vi "HEWH Mixing Valve.vi"(8 "Error In":errorcluster, 10 "ERD Data Out":T4[](array[typedef]) {"ERD Number" format="%.0x"}, 11 "ERD Data":T1 {"ERD Therm Data"."EEV Possition" format="%0.0f"; "ERD Therm Data"."T6" format="%.1f"; "ERD Therm Data"."T2" format="%.1f"; "ERD Therm Data"."T3a" format="%.1f"; "ERD Therm Data"."T3b" format="%.1f"; "ERD Therm Data"."T4" format="%.1f"; "ERD Therm Data"."T5" format="%.1f"; "ERD Therm Data"."Current" format="%.1f"}) -> (0 "Error Out":errorcluster, 3 "ERD Data Out":T1 {"ERD Therm Data"."EEV Possition" format="%0.0f"; "ERD Therm Data"."T6" format="%.1f"; "ERD Therm Data"."T2" format="%.1f"; "ERD Therm Data"."T3a" format="%.1f"; "ERD Therm Data"."T3b" format="%.1f"; "ERD Therm Data"."T4" format="%.1f"; "ERD Therm Data"."T5" format="%.1f"; "ERD Therm Data"."Current" format="%.1f"})   [LabVIEW 2016]
uses:
  type defs/ERD Read Data Out.ctl
  type defs/HEWH ERD Data.ctl
  type defs/HEWH Faults.ctl
  type defs/HEWH Mixing Valve.ctl
  library/GEA2_Toolkit.lvlib
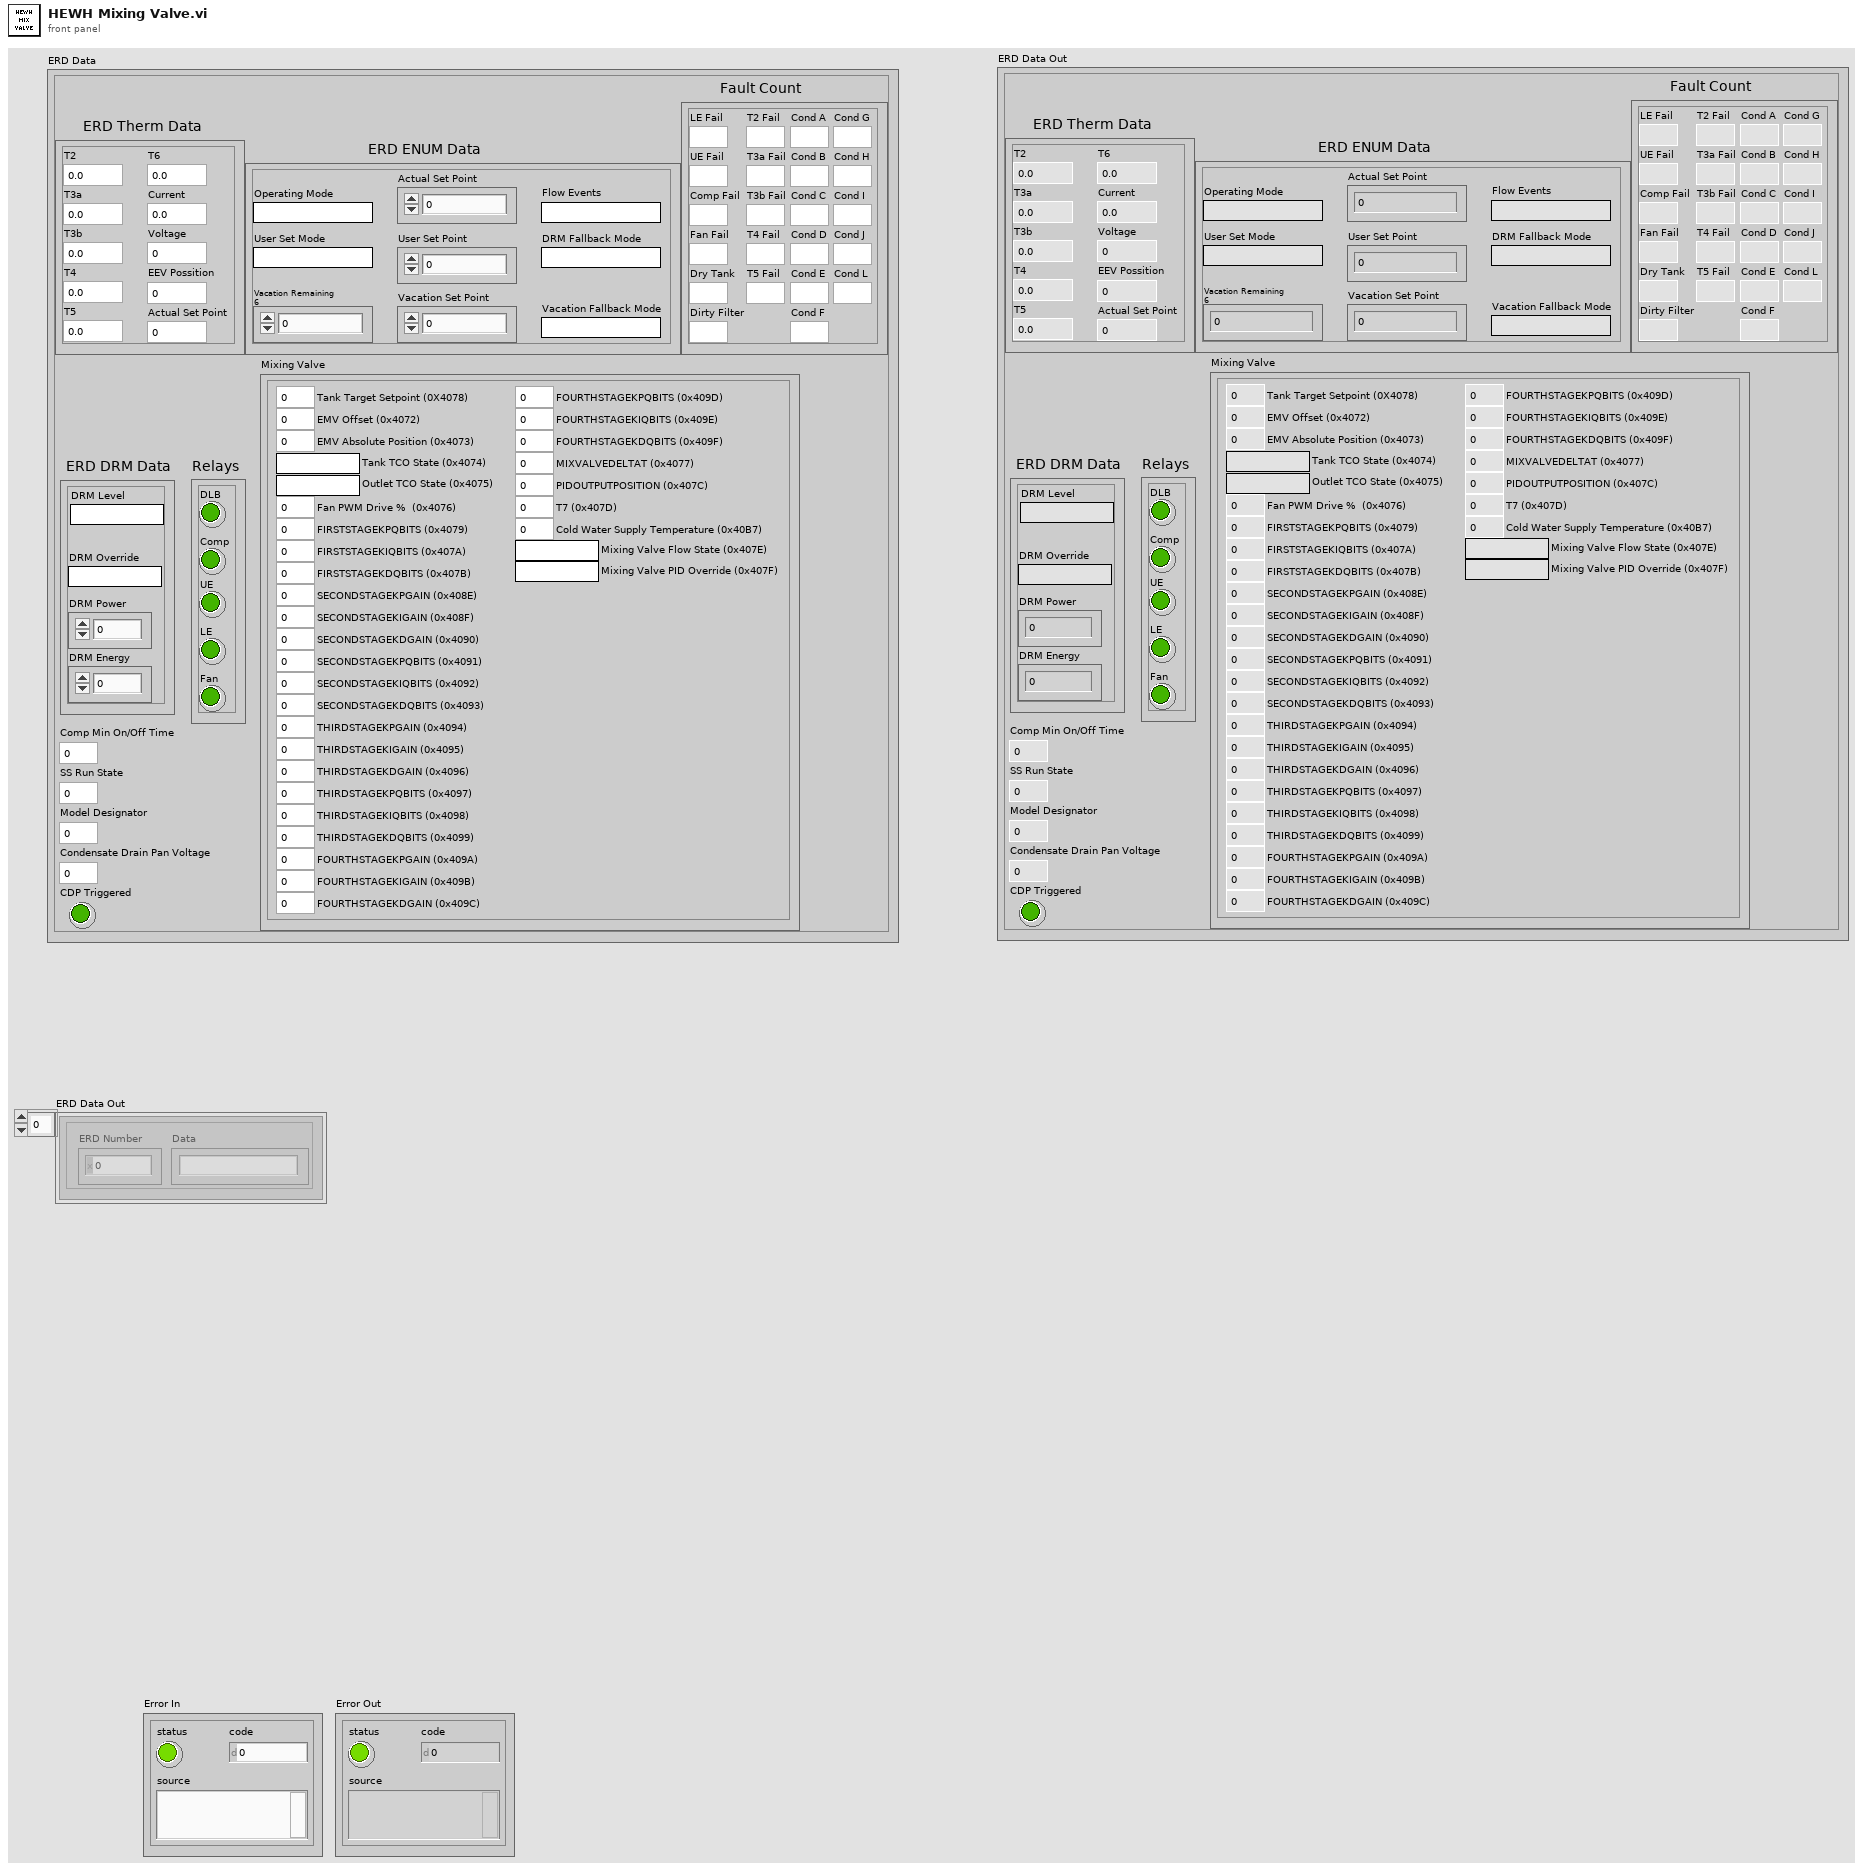
[diagram p1: front panel]
types:
  T1 = typedef "HEWH ERD Data.ctl" = cluster{"ERD Therm Data":cluster{"T2":dbl, "T3a":dbl, "T3b":dbl, "T4":dbl, "T5":dbl, "T6":dbl, "Current":dbl, "Voltage":dbl, "EEV Possition":dbl, "Actual Set Point":dbl}, "ERD ENUM Data":cluster{"Actual Set Point":dbl, "Flow Events":string, "User Set Mode":string, "Operating Mode":string, "DRM Fallback Mode":string, "Vacation Fallback Mode":string, "User Set Point":dbl, "Vacation Set Point":dbl, "Vacation Remaining\n6":dbl}, "ERD DRM Data":cluster{"DRM Level":string, "DRM Override":string, "DRM Power":dbl, "DRM Energy":dbl}, "Fault Count":T2, "Relays":cluster{"DLB":bool, "Comp":bool, "UE":bool, "LE":bool, "Fan":bool}, "Comp Min On/Off Time":u16, "SS Run State":u16, "Condensate Drain Pan Voltage":u16, "CDP Triggered":bool, "Model Designator":u8, "Mixing Valve":T3}
  T2 = typedef "HEWH Faults.ctl" = cluster{"LE Fail":u32, "UE Fail":u32, "Comp Fail":u32, "T2 Fail":u32, "T3a Fail":u32, "T3b Fail":u32, "T4 Fail":u32, "T5 Fail":u32, "Cond A":u32, "Cond B":u32, "Cond C":u32, "Cond D":u32, "Cond E":u32, "Cond F":u32, "Cond G":u32, "Cond H":u32, "Cond I":u32, "Cond J":u32, "Cond L":u32, "Fan Fail":u32, "Dirty Filter":u32, "Dry Tank":u32}
  T3 = typedef "HEWH Mixing Valve.ctl" = cluster{"Tank Target Setpoint (0X4078)":dbl, "EMV Offset (0x4072)":dbl, "EMV Absolute Position (0x4073)":dbl, "Tank TCO State (0x4074)":string, "Outlet TCO State (0x4075)":string, "Fan PWM Drive %  (0x4076)":dbl, "FIRSTSTAGEKPQBITS (0x4079)":dbl, "FIRSTSTAGEKIQBITS (0x407A)":dbl, "FIRSTSTAGEKDQBITS (0x407B)":dbl, "SECONDSTAGEKPGAIN (0x408E)":dbl, "SECONDSTAGEKIGAIN (0x408F)":dbl, "SECONDSTAGEKDGAIN (0x4090)":dbl, "SECONDSTAGEKPQBITS (0x4091)":dbl, "SECONDSTAGEKIQBITS (0x4092)":dbl, "SECONDSTAGEKDQBITS (0x4093)":dbl, "THIRDSTAGEKPGAIN (0x4094)":dbl, "THIRDSTAGEKIGAIN (0x4095)":dbl, "THIRDSTAGEKDGAIN (0x4096)":dbl, "THIRDSTAGEKPQBITS (0x4097)":dbl, "THIRDSTAGEKIQBITS (0x4098)":dbl, "THIRDSTAGEKDQBITS (0x4099)":dbl, "FOURTHSTAGEKPGAIN (0x409A)":dbl, "FOURTHSTAGEKIGAIN (0x409B)":dbl, "FOURTHSTAGEKDGAIN (0x409C)":dbl, "FOURTHSTAGEKPQBITS (0x409D)":dbl, "FOURTHSTAGEKIQBITS (0x409E)":dbl, "FOURTHSTAGEKDQBITS (0x409F)":dbl, "MIXVALVEDELTAT (0x4077)":dbl, "PIDOUTPUTPOSITION (0x407C)":dbl, "T7 (0x407D)":dbl, "Cold Water Supply Temperature (0x40B7)":dbl, "Mixing Valve Flow State (0x407E)":string, "Mixing Valve PID Override (0x407F)":string}
  T4 = typedef "GEA2_Toolkit.lvlib/ERD Read Data Out.ctl" = cluster{"ERD Number":u16, "Data":string}
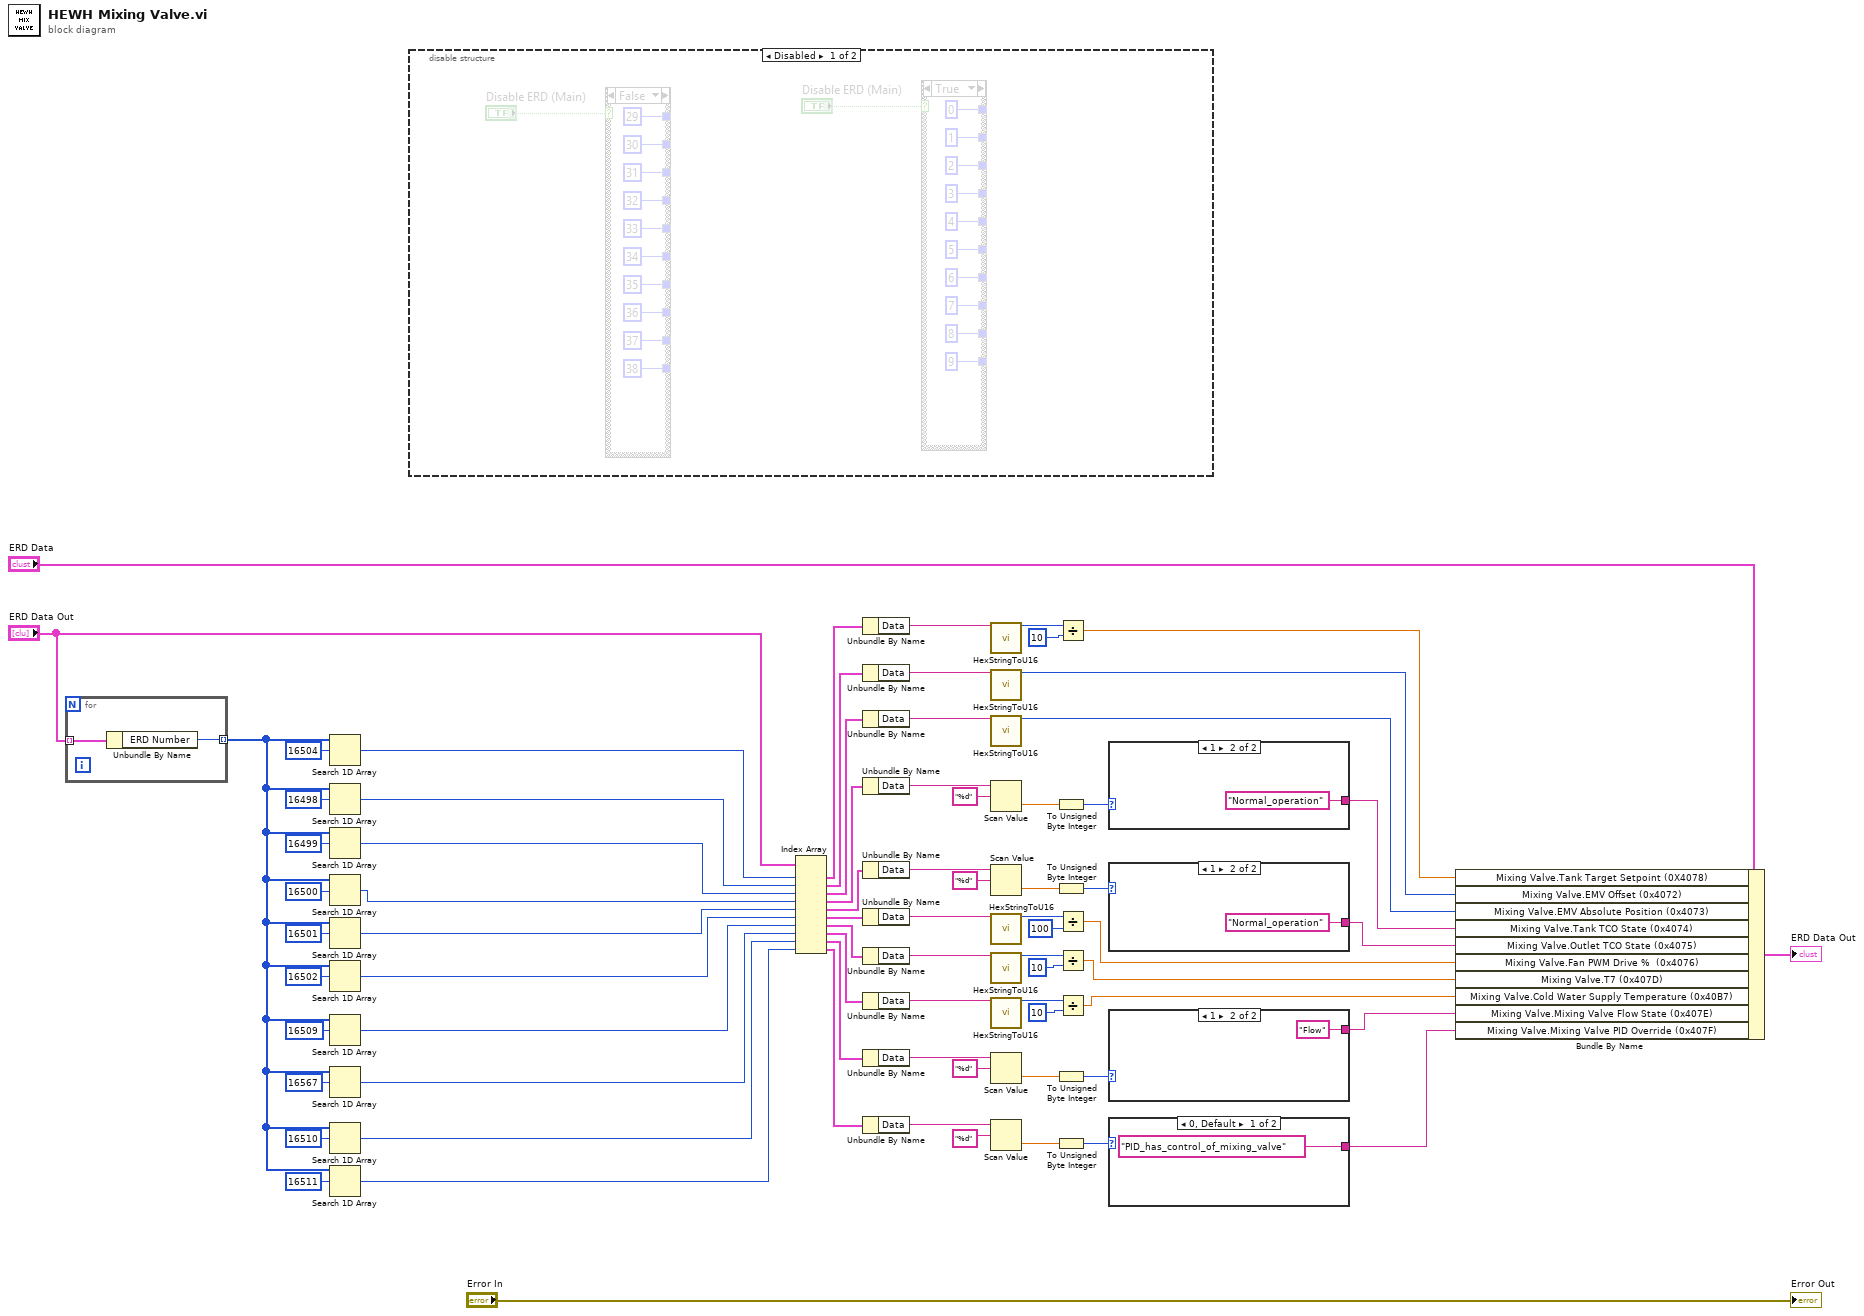
[diagram p0: block diagram]
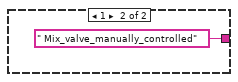
[diagram p3: hidden frame]
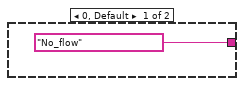
[diagram p4: hidden frame]
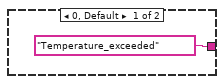
[diagram p5: hidden frame]
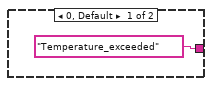
[diagram p6: hidden frame]
diagram:
  n1 = for {
    tunnel: "ERD Data Out" -> [w77] mode=indexing
    tunnel: [w76] -> w11 mode=indexing
    n2 = Unbundle By Name(w77) -> ("ERD Number"=w76:u16)
  }
  n3 = Search 1D Array(1D array=w11, element=u16 16504 ("ERD Number")) -> (index of element=w10:i32)  [unwired: 1 in]
  n4 = Search 1D Array(1D array=w11, element=u16 16498 ("ERD Number")) -> (index of element=w9:i32)  [unwired: 1 in]
  n5 = Search 1D Array(1D array=w11, element=u16 16499 ("ERD Number")) -> (index of element=w8:i32)  [unwired: 1 in]
  n6 = Search 1D Array(1D array=w11, element=u16 16500 ("ERD Number")) -> (index of element=w7:i32)  [unwired: 1 in]
  n7 = Search 1D Array(1D array=w11, element=u16 16501 ("ERD Number")) -> (index of element=w6:i32)  [unwired: 1 in]
  n8 = Search 1D Array(1D array=w11, element=u16 16502 ("ERD Number")) -> (index of element=w5:i32)  [unwired: 1 in]
  n9 = Search 1D Array(1D array=w11, element=u16 16509 ("ERD Number")) -> (index of element=w4:i32)  [unwired: 1 in]
  n10 = Search 1D Array(1D array=w11, element=u16 16567 ("ERD Number")) -> (index of element=w3:i32)  [unwired: 1 in]
  n11 = Search 1D Array(1D array=w11, element=u16 16510 ("ERD Number")) -> (index of element=w2:i32)  [unwired: 1 in]
  n12 = Search 1D Array(1D array=w11, element=u16 16511 ("ERD Number")) -> (index of element=w1:i32)  [unwired: 1 in]
  n13 = disable-structure shown="Disabled" {
    frame Disabled {
    }
    frame Enabled {
    }
  }
  n14 = Index Array(array="ERD Data Out", index #1=w10, index #2=w9, index #3=w8, index #4=w7, index #5=w6, index #6=w5, index #7=w4, index #8=w3, index #9=w2, index #10=w1) -> (element #1=w75:T4, element #2=w74:T4, element #3=w73:T4, element #4=w72:T4, element #5=w71:T4, element #6=w70:T4, element #7=w65:T4, element #8=w64:T4, element #9=w63:T4, element #10=w59:T4)
  n15 = Unbundle By Name(w75) -> ("Data"=w55:string)
  n16 = Unbundle By Name(w74) -> ("Data"=w53:string)
  n17 = Unbundle By Name(w73) -> ("Data"=w51:string)
  n18 = Unbundle By Name(w72) -> ("Data"=w48:string)
  n19 = Unbundle By Name(w71) -> ("Data"=w44:string)
  n20 = Unbundle By Name(w70) -> ("Data"=w40:string)
  n21 = Unbundle By Name(w65) -> ("Data"=w36:string)
  n22 = Unbundle By Name(w64) -> ("Data"=w32:string)
  n23 = Unbundle By Name(w63) -> ("Data"=w28:string)
  n24 = Unbundle By Name(w59) -> ("Data"=w24:string)
  n25 = call "HexStringToU16.vi"("Input String"=w55) -> ("Number Out"=w56:u16)  [unwired: 14 in]
  n26 = call "HexStringToU16.vi"("Input String"=w53) -> ("Number Out"=w52:u16)  [unwired: 14 in]
  n27 = call "HexStringToU16.vi"("Input String"=w51) -> ("Number Out"=w50:u16)  [unwired: 14 in]
  n28 = Scan Value(string=w48, format string="%d") -> (value=w49:dbl)  [unwired: 1 in, 1 out]
  n29 = Scan Value(string=w44, format string="%d") -> (value=w46:dbl)  [unwired: 1 in, 1 out]
  n30 = call "HexStringToU16.vi"("Input String"=w40) -> ("Number Out"=w42:u16)  [unwired: 14 in]
  n31 = call "HexStringToU16.vi"("Input String"=w36) -> ("Number Out"=w38:u16)  [unwired: 14 in]
  n32 = call "HexStringToU16.vi"("Input String"=w32) -> ("Number Out"=w33:u16)  [unwired: 14 in]
  n33 = Scan Value(string=w28, format string="%d") -> (value=w30:dbl)  [unwired: 1 in, 1 out]
  n34 = Scan Value(string=w24, format string="%d") -> (value=w25:dbl)  [unwired: 1 in, 1 out]
  n35 = To Unsigned Byte Integer(number=w49) -> (unsigned 8bit integer=w47:u8)
  n36 = To Unsigned Byte Integer(number=w46) -> (unsigned 8bit integer=w43:u8)
  n37 = To Unsigned Byte Integer(number=w30) -> (unsigned 8bit integer=w27:u8)
  n38 = To Unsigned Byte Integer(number=w25) -> (unsigned 8bit integer=w23:u8)
  n39 = Divide(x=w56, y=u16 10) -> (x/y=w54:dbl)
  n40 = Divide(x=w42, y=u16 100) -> (x/y=w39:dbl)
  n41 = Divide(x=w38, y=u16 10) -> (x/y=w35:dbl)
  n42 = Divide(x=w33, y=u16 10) -> (x/y=w31:dbl)
  n43 = case shown="1" w47 {
    tunnel: ["Temperature_exceeded" "Normal_operation"] -> w69
    frame 0, Default {
    }
    frame 1 {
    }
  }
  n44 = case shown="1" w43 {
    tunnel: ["Temperature_exceeded" "Normal_operation"] -> w68
    frame 0, Default {
    }
    frame 1 {
    }
  }
  n45 = case shown="1" w27 {
    tunnel: ["No_flow" "Flow"] -> w67
    frame 0, Default {
    }
    frame 1 {
    }
  }
  n46 = case shown="0, Default" w23 {
    tunnel: ["PID_has_control_of_mixing_valve" " Mix_valve_manually_controlled"] -> w66
    frame 0, Default {
    }
    frame 1 {
    }
  }
  n47 = Bundle By Name(cluster="ERD Data", "Mixing Valve.Tank Target Setpoint (0X4078)"=w54, "Mixing Valve.EMV Offset (0x4072)"=w52, "Mixing Valve.EMV Absolute Position (0x4073)"=w50, "Mixing Valve.Tank TCO State (0x4074)"=w69, "Mixing Valve.Outlet TCO State (0x4075)"=w68, "Mixing Valve.Fan PWM Drive %  (0x4076)"=w39, "Mixing Valve.T7 (0x407D)"=w35, "Mixing Valve.Cold Water Supply Temperature (0x40B7)"=w31, "Mixing Valve.Mixing Valve Flow State (0x407E)"=w67, "Mixing Valve.Mixing Valve PID Override (0x407F)"=w66) -> (→"ERD Data Out":T1)
  "Error Out" <- "Error In"
